vi "read save configuration file.vi"(7 "VI Reference":refnum<vi>, 8 "error in (no error)":errorcluster, 9 "Write Ini":bool, 10 "Read Ini":bool, 11 "Path":path=path "C:/Users/CWEDD/Documents/LabVIEW Data/Waterloo DAQ/config files/DAQ Setup Config.ini") -> (0 "error out":errorcluster)   [LabVIEW 2016]
uses:
  <vilib>/Utility/config.llb/NI_LVConfig.lvlib
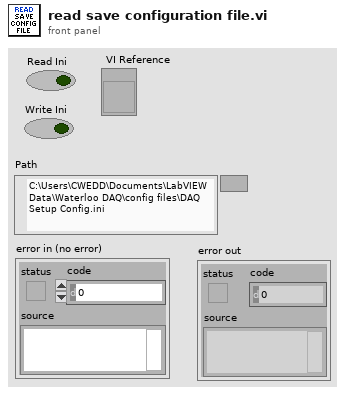
[diagram p1: front panel]
types:
  T1 = typedef "NI_LVConfig.lvlib/Config Data RefNum.ctl" = refnum<k1>
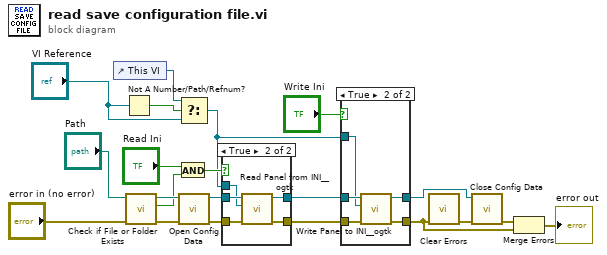
[diagram p0: block diagram]
diagram:
  n1 = control-ref of="This VI"() -> (w3:refnum<vi>)
  n2 = Not A Number/Path/Refnum?(number/path/refnum="VI Reference") -> (NaN/Path/Refnum?=w2:bool)
  n3 = call <vilib>:"Check if File or Folder Exists.vi"("error in (no error)"="error in (no error)", "path"="Path") -> ("error out"=w17:errorcluster, "file or folder exists?"=w5:bool, "dup path"=w18:path)  [unwired: 7 in]
  n4 = And(x="Read Ini", y=w5) -> (x .and. y?=w6:bool)
  n5 = Select(t=w3, s=w2, f="VI Reference") -> (s? t:f=w4:refnum<vi>)
  n6 = call <vilib>:"Open Config Data.vi"("error in (no error)"=w17, "configuration file path"=w18) -> ("error out"=w15:errorcluster, "refnum"=w16:T1)  [unwired: 7 in, 1 out]
  n7 = case shown="True" w6 {
    tunnel: w16 -> [w23 w28]
    tunnel: w15 -> [w22 w27]
    tunnel: w4 -> [_ w26]
    tunnel: [w22 w25] -> w10
    tunnel: [w23 w24] -> w11
    frame False {
    }
    frame True {
      n8 = call "Read Panel from INI__ogtk.vi"("error in (no error)"=w27, "VI ref"=w26, "refnum"=w28) -> ("error out"=w25:errorcluster, "refnum out"=w24:T1)  [unwired: 7 in]
    }
  }
  n9 = case shown="True" "Write Ini" {
    tunnel: w11 -> [w30 w35]
    tunnel: w10 -> [w29 w34]
    tunnel: w4 -> [_ w33]
    tunnel: [w30 w32] -> w9
    tunnel: [w29 w31] -> w8
    frame False {
    }
    frame True {
      n10 = call "Write Panel to INI__ogtk.vi"("error in (no error)"=w34, "VI ref"=w33, "refnum"=w35) -> ("error out"=w31:errorcluster, "refnum out"=w32:T1)  [unwired: 7 in]
    }
  }
  n11 = call <vilib>:"Clear Errors.vi"("error in (no error)"=w8) -> ("error out"=w14:errorcluster)  [unwired: 5 in, 1 out]
  n12 = call <vilib>:"Close Config Data.vi"("error in (no error)"=w14, "refnum"=w9) -> ("error out"=w13:errorcluster)  [unwired: 8 in, 1 out]
  n13 = Merge Errors(w13, w8) -> (→"error out":errorcluster)
